vi "Load Bitfile.vi"() -> ()   [LabVIEW 2011, in "LVH-Adept.lvlib"]
uses:
  <vilib>/LabVIEW Hacker/Adept/LVH-Adept.lvlib
  <vilib>/LabVIEW Hacker/Adept/Private/Type Defs/Adept Device Ctl.xctl
panel:
  in  "Bit File Path":path
  in  "Adept Device":u16(xcontrol)
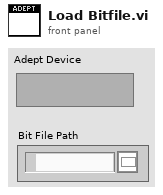
[diagram p1: front panel]
types:
  T1 = typedef "LVH-Adept.lvlib/Device Config.ctl" = cluster{"Num Devices":i32, "Device Names":string[], "Device Index":u16, "Device Handle":u32}
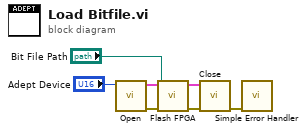
[diagram p0: block diagram]
diagram:
  n1 = call <vilib>:"Open.vi"("Adept Device Ctl"="Adept Device") -> ("Error Out"=w6:errorcluster, "Adept Config"=w7:T1)  [unwired: 9 in]
  n2 = call <vilib>:"Flash FPGA.vi"("Error In"=w6, "Bit File Path"="Bit File Path", "Adept Config"=w7) -> ("Error Out"=w5:errorcluster, "Adept Config"=w4:T1)  [unwired: 7 in]
  n3 = call <vilib>:"Close.vi"("Error In"=w5, "Adept Config"=w4) -> ("Error Out"=w2:errorcluster)  [unwired: 9 in]
  n4 = call <vilib>:"Simple Error Handler.vi"("error in (no error)"=w2) -> ()  [unwired: 4 in, 5 out]
